vi "Initialise Cubes.vi"(8 "error in (no error)":errorcluster, 10 "Number Of Cubes":i32=10, 11 "Resource Directory":path) -> (0 "error out":errorcluster, 3 "Cubes":T1[](array[typedef]))   [LabVIEW 2022 SP3, in "Application.lvlib" / "Scene.lvclass"]
uses:
  Scene.lvclass
  Libraries/3D/Object.ctl
  Libraries/3D/Triangle 3D.ctl
  Libraries/3D/Vector 3D.ctl
  Libraries/3D/Transform.ctl
  <vilib>/numeric/Random Number (Range) DBL.vi
  Libraries/3D/3D.lvlib
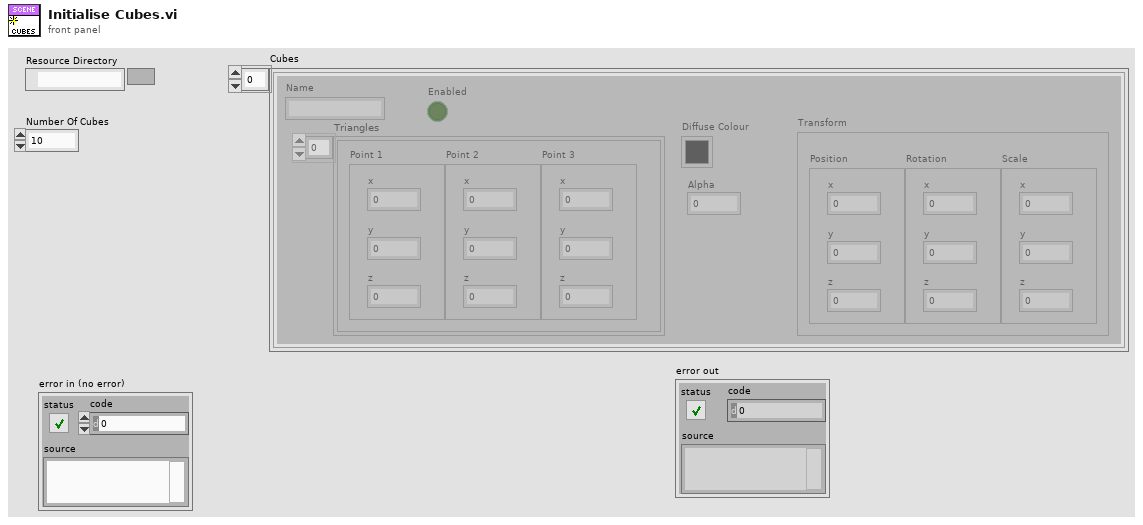
[diagram p1: front panel]
types:
  T1 = typedef "3D.lvlib/Object.ctl" = cluster{"Triangles":T2[], "Diffuse Colour":u32, "Transform":T4, "Name":string, "Enabled":bool, "Alpha":dbl}
  T2 = typedef "3D.lvlib/Triangle 3D.ctl" = cluster{"Point 1":T3, "Point 2":T3, "Point 3":T3}
  T3 = typedef "3D.lvlib/Vector 3D.ctl" = cluster{"x":sgl, "y":sgl, "z":sgl}
  T4 = typedef "3D.lvlib/Transform.ctl" = cluster{"Position":T3, "Rotation":T3, "Scale":T3}
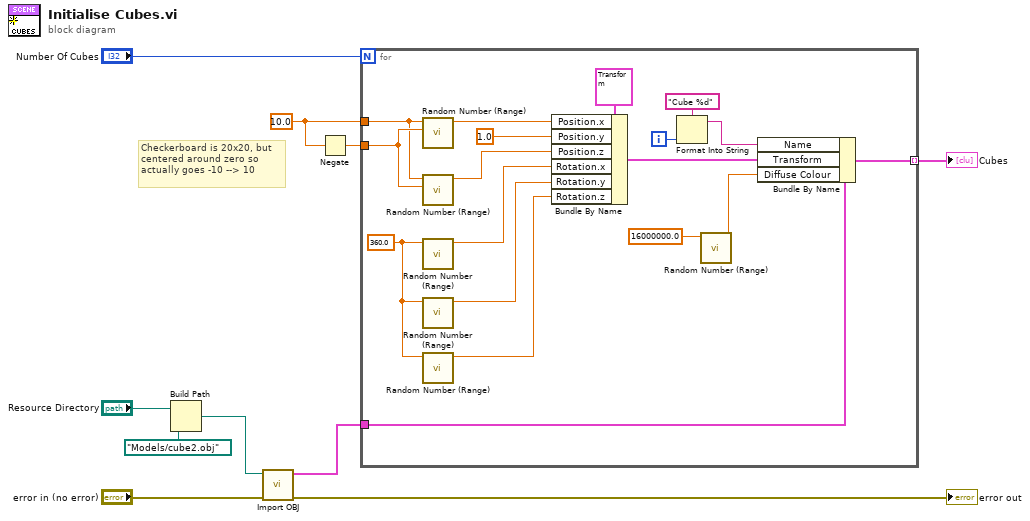
[diagram p0: block diagram]
diagram:
  w5 = 10.0 ("upper bound (100)")
  # "Checkerboard is 20x20, but centered around zero so actually goes -10 --> 10"
  n1 = Build Path(base path="Resource Directory", name or relative path=path "Models/cube2.obj") -> (appended path=w8:path)
  n2 = call "Import OBJ.vi"("error in (no error)"="error in (no error)", "Object"=w8) -> ("error out"=→"error out":errorcluster, "Object"=w10:T1)  [unwired: 8 in]
  n3 = Negate(x=w5) -> (-x=w4:dbl)
  n4 = for {
    N: "Number Of Cubes" -> [_]
    tunnel: w10 -> [w28]
    tunnel: [w24] -> w6 mode=indexing
    tunnel: w5 -> [w17]
    tunnel: w4 -> [w18]
    i -> [w21]
    w13 = 360.0 ("upper bound (100)")
    n5 = call-poly <vilib>:"Random Number (Range).vi"("lower bound (0)"=w18, "upper bound (100)"=w17) -> ("number"=w20:dbl)  [unwired: 9 in]
    n6 = call-poly <vilib>:"Random Number (Range).vi"("lower bound (0)"=w18, "upper bound (100)"=w17) -> ("number"=w19:dbl)  [unwired: 9 in]
    n7 = call-poly <vilib>:"Random Number (Range).vi"("upper bound (100)"=w13) -> ("number"=w14:dbl)  [unwired: 10 in]
    n8 = call-poly <vilib>:"Random Number (Range).vi"("upper bound (100)"=w13) -> ("number"=w12:dbl)  [unwired: 10 in]
    n9 = call-poly <vilib>:"Random Number (Range).vi"("upper bound (100)"=w13) -> ("number"=w11:dbl)  [unwired: 10 in]
    n10 = Bundle By Name(cluster=T4 {"Position"={"x"=2.0, "y"=1.0, "z"=-5.0}, "Rotation"={"x"=0.0, "y"=0.0, "z"=0.0}, "Scale"={"x"=0.0, "y"=0.0, "z"=0.0}} ("Transform"), "Position.x"=w20, "Position.y"=sgl 1.0, "Position.z"=w19, "Rotation.x"=w14, "Rotation.y"=w12, "Rotation.z"=w11) -> (w26:T4)
    n11 = Format Into String(format string="Cube %d" ("Name"), w21) -> (resulting string=w22:string)  [unwired: 2 in, 1 out]
    n12 = call-poly <vilib>:"Random Number (Range).vi"("upper bound (100)"=16000000.0) -> ("number"=w15:dbl)  [unwired: 10 in]
    n13 = Bundle By Name(cluster=w28, "Name"=w22, "Transform"=w26, "Diffuse Colour"=w15) -> (w24:T1)
  }
  "Cubes" <- w6
